vi "PH_ImageOperator.Reduce Fit Trace.vi"(2 "Diameter":dbl, 7 "Best Fit Trace":cluster{"Index":sgl[], "Best Fit":dbl[]}) -> (8 "Reduced Best Fit Trace":cluster{"Index":sgl[], "Best Fit":dbl[]})   [LabVIEW 2014, in "PH_ImageOperator.lvlib"]
doc: "This VI reduces the trace entries to a third of the origional amount of data to speed up the fit procedure. It also reduces the trace to 4 times of the \"diameter\"."
uses:
  PH_ImageOperator.lvlib
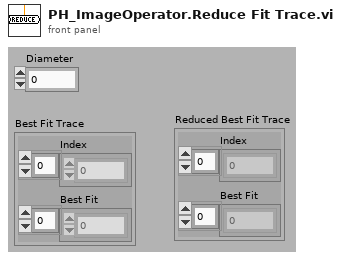
[diagram p1: front panel]
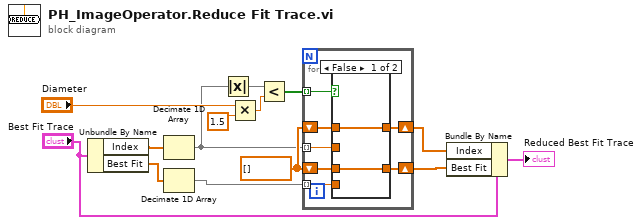
[diagram p0: block diagram]
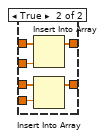
[diagram p2: hidden frame]
diagram:
  w7 = sgl[] []
  n1 = Unbundle By Name("Best Fit Trace") -> ("Index"=w14:sgl[], "Best Fit"=w13:dbl[])
  n2 = Decimate 1D Array(w14) -> (w4:sgl[])  [unwired: 2 out]
  n3 = Decimate 1D Array(w13) -> (w3:dbl[])  [unwired: 2 out]
  n4 = Absolute Value(x=w4) -> (abs(x)=w10:sgl[])
  n5 = Multiply(x="Diameter", y=1.5) -> (x*y=w9:dbl)
  n6 = Less?(x=w10, y=w9) -> (x < y?=w8:bool[])
  n7 = for {
    tunnel: w4 -> [w20] mode=indexing
    tunnel: w3 -> [w16] mode=indexing
    tunnel: w8 -> [w15] mode=indexing
    shift-right: [w19] -> w2
    shift-left: w7 -> [w21]
    shift-right: [w17] -> w1
    shift-left: w7 -> [w18]
    n8 = case shown="False" w15 {
      tunnel: w21 -> [w23 w29]
      tunnel: w20 -> [_ w25]
      tunnel: [w23 w28] -> w19
      tunnel: w18 -> [w22 w27]
      tunnel: [w22 w26] -> w17
      tunnel: w16 -> [_ w24]
      frame False {
      }
      frame True {
        n9 = Insert Into Array(array=w29, new element=w25) -> (w28:sgl[])  [unwired: 1 in]
        n10 = Insert Into Array(array=w27, new element=w24) -> (w26:sgl[])  [unwired: 1 in]
      }
    }
  }
  n11 = Bundle By Name(cluster="Best Fit Trace", "Index"=w2, "Best Fit"=w1) -> (→"Reduced Best Fit Trace":cluster{"Index":sgl[], "Best Fit":dbl[]})
